vi "joystick+serial to robot.vi"() -> ()   [LabVIEW 2016]
uses:
  grSim Robot Command.ctl
  <vilib>/Instr/_visa.llb/VISA Configure Serial Port (Instr).vi
panel:
  out "Numeric 2":dbl
  out "String":string
  out "output cluster":T1
  out "return count":u32
  in  "stop":bool
  out "string":string
  out "error out":errorcluster
  in  "termination char\n(0xA = '\\n' = LF)":u8=10 format="%.0x"
  in  "VISA resource name":refnum<visa-resource-name>
  in  "Serial Settings":T2={"baud rate"=9600, "data bits"=8, "parity"=enum."None", "stop bits"=10, "flow control"=0} {"flow control" items=["None"=0, "XON/XOFF"=1, "RTS/CTS"=2, "DTR/DSR"=4]; "stop bits" items=["1.0"=10, "1.5"=15, "2.0"=20]; "data bits" min=5 max=8 step=1; "baud rate" items=["75"=75, "110"=110, "134"=134, "150"=150, "300"=300, "600"=600, "1200"=1200, "1800"=1800, "2400"=2400, "4800"=4800, "7200"=7200, "9600"=9600, "14400"=14400, "19200"=19200, "28800"=28800, "38400"=38400, "56000"=56000, "57600"=57600, "115200"=115200, "128000"=128000, "230400"=230400]}
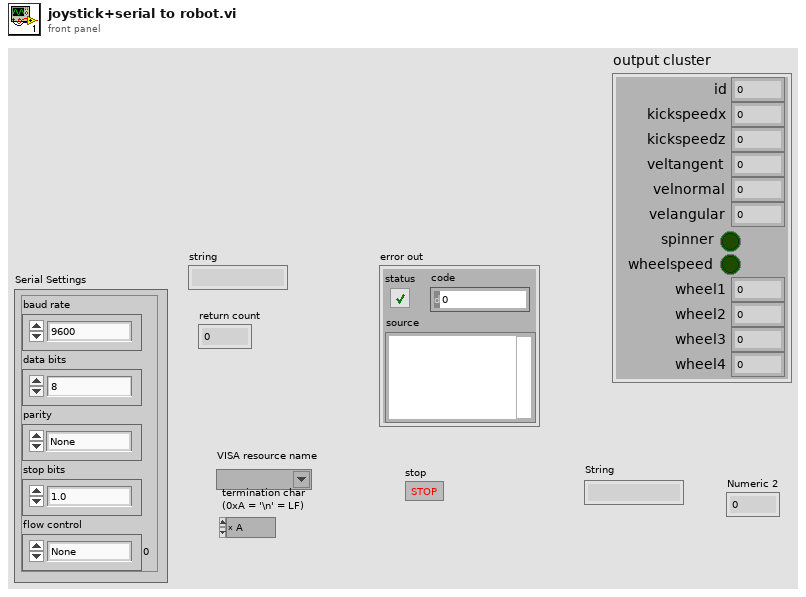
[diagram p1: front panel]
types:
  T1 = typedef "grSim Robot Command.ctl" = cluster{"id":u32, "kickspeedx":sgl, "kickspeedz":sgl, "veltangent":sgl, "velnormal":sgl, "velangular":sgl, "spinner":bool, "wheelspeed":bool, "wheel1":sgl, "wheel2":sgl, "wheel3":sgl, "wheel4":sgl}
  T2 = cluster{"baud rate":u32, "data bits":u16, "parity":enum16{"None", "Odd", "Even", "Mark", "Space"}, "stop bits":u16, "flow control":u16}
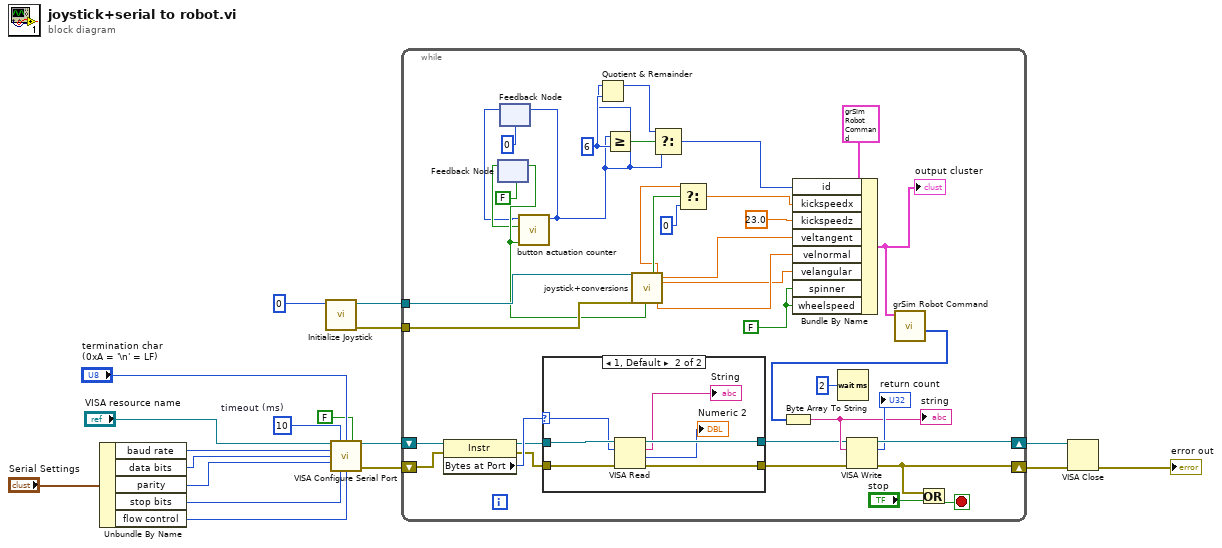
[diagram p0: block diagram]
diagram:
  w4 = u32 10  # timeout (ms)
  n1 = Unbundle By Name("Serial Settings") -> ("baud rate"=w17:u32, "data bits"=w16:u16, "parity"=w15:enum16{"None", "Odd", "Even", "Mark", "Space"}, "stop bits"=w14:u16, "flow control"=w13:u16)
  n2 = call <vilib>:"Initialize Joystick.vi"("device index"=0) -> ("error out"=w1:errorcluster, "device ID"=w2:refnum<k1>)  [unwired: 9 in]
  n3 = call-poly "VISA Configure Serial Port"("VISA resource name"="VISA resource name", "timeout (10sec)"=w4, "termination char\n(0xA = '\\n' = LF)"="termination char\n(0xA = '\\n' = LF)", "Enable Termination\nChar (T)"=FALSE ("Enable Termination\nChar (T)"), "baud rate (9600)"=w17, "data bits (8)"=w16, "parity (0:none)"=w15, "stop bits (10: 1 bit)"=w14, "flow control (0:none)"=w13) -> ("VISA resource name out"=w9:refnum<visa-resource-name>, "error out"=w7:errorcluster)  [unwired: 5 in]
  n4 = while {
    shift-right: [w56] -> w8
    shift-left: w9 -> [w23]
    shift-right: [w52] -> w6
    shift-left: w7 -> [w22]
    tunnel: w2 -> [w42]
    tunnel: w1 -> [w41]
    stop <- w53 stop-if-true
    w37 = 6 ("y")
    w43 = FALSE
    n5 = property class="Instr"(reference=w23, error in=w22) -> (reference out=w19:refnum<visa-resource-name>, error out=w20:errorcluster, "Bytes at Port"=w21:u32)
    n6 = feedback #1(FALSE) -> (w34:bool)
    n7 = feedback #2(0) -> (w31:i32)
    n8 = case shown="1, Default" w21 {
      selector: w21 -> [_ w59]
      tunnel: w20 -> [w57 w65]
      tunnel: [w57 w64] -> w25
      tunnel: w19 -> [w58 w63]
      tunnel: [w58 w62] -> w24
      frame 0 {
      }
      frame 1, Default {
        n9 = VISA Read(VISA resource name=w63, byte count=w59, error in (no error)=w65) -> (VISA resource name out=w62:refnum<visa-resource-name>, read buffer=→"String":string, return count=→"Numeric 2":u32, error out=w64:errorcluster)
      }
    }
    n10 = call "joystick+conversions.vi"("Refnum in"=w42, "error in (no error)"=w41) -> ("B pressed"=w35:bool, "v_radial"=w44:dbl, "A pressed"=w28:bool, "chute"=w26:dbl, "v_normal"=w46:dbl, "R*w"=w45:dbl)  [unwired: 9 in, 11 out]
    n11 = feedback-in #1(w35) -> ()
    n12 = call "button actuation counter.vi"("old count"=w31, "was button pressed ?"=w34, "button pressed now"=w35) -> ("new count"=w32:i32)  [unwired: 7 in]
    n13 = feedback-in #2(w32) -> ()
    n14 = Quotient & Remainder(x=w32, y=w37) -> (x-y*floor(x/y)=w36:i32)  [unwired: 1 out]
    n15 = Greater Or Equal?(x=w32, y=w37) -> (x >= y?=w39:bool)
    n16 = Select(t=w36, s=w39, f=w32) -> (s? t:f=w38:i32)
    n17 = Select(t=w26, s=w28, f=0) -> (s? t:f=w27:dbl)
    n18 = Bundle By Name(cluster=T1 {"id"=0, "kickspeedx"=0.0, "kickspeedz"=0.0, "veltangent"=0.0, "velnormal"=0.0, "velangular"=0.0, "spinner"=FALSE, "wheelspeed"=FALSE, "wheel1"=0.0, "wheel2"=0.0, "wheel3"=0.0, "wheel4"=0.0} ("Robots"), "id"=w38, "kickspeedx"=w27, "kickspeedz"=sgl 23.0 ("kickspeedx"), "veltangent"=w44, "velnormal"=w46, "velangular"=w45, "spinner"=w43, "wheelspeed"=w43) -> (w40:T1)
    "output cluster" <- w40
    n19 = Wait (ms)(milliseconds to wait=u32 2) -> ()  [unwired: 1 out]
    n20 = call "grSim Robot Command.vi"("Robots"=w40) -> ("Array"=w49:u8[])  [unwired: 10 in]
    n21 = Byte Array To String(unsigned byte array=w49) -> (string=w50:string)
    "string" <- w50
    n22 = VISA Write(VISA resource name=w24, write buffer=w50, error in (no error)=w25) -> (VISA resource name out=w56:refnum<visa-resource-name>, return count=→"return count":u32, error out=w52:errorcluster)
    n23 = Or(x=w52, y="stop") -> (x .or. y?=w53:bool)
  }
  n24 = VISA Close(VISA resource name=w8, error in (no error)=w6) -> (error out=→"error out":errorcluster)
